vi "Random Graph Generator.vi"() -> ()   [LabVIEW 2021]
panel:
  in  "Array":T1(array[cluster])
  in  "Show Graph?":bool
  in  "Graph Type":enum16{"Velocity", "Position"}(ring)=enum."Position"
  out "Waveform Graph":dbl[][](graph)
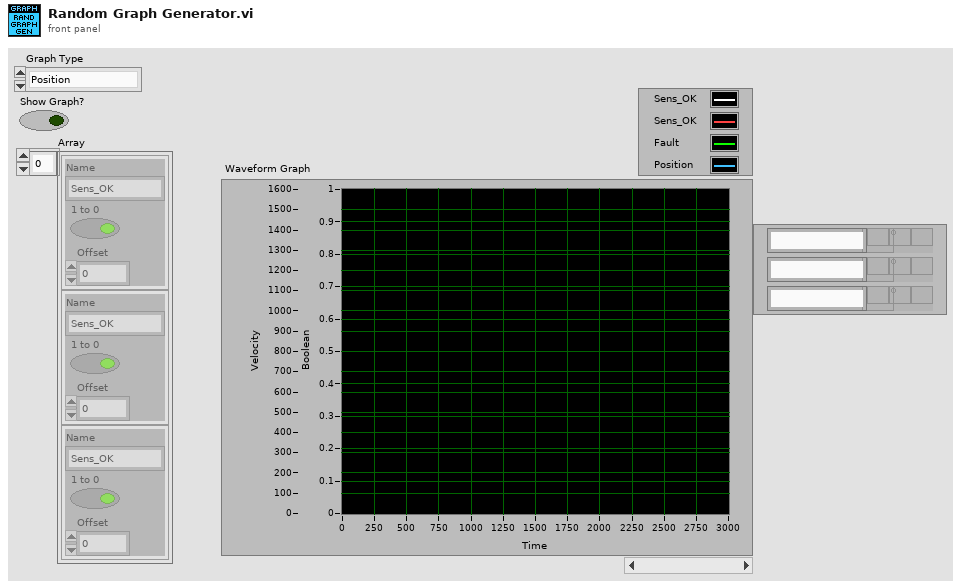
[diagram p1: front panel]
types:
  T1 = cluster{"Name":string, "1 to 0":bool, "Offset":dbl}[]
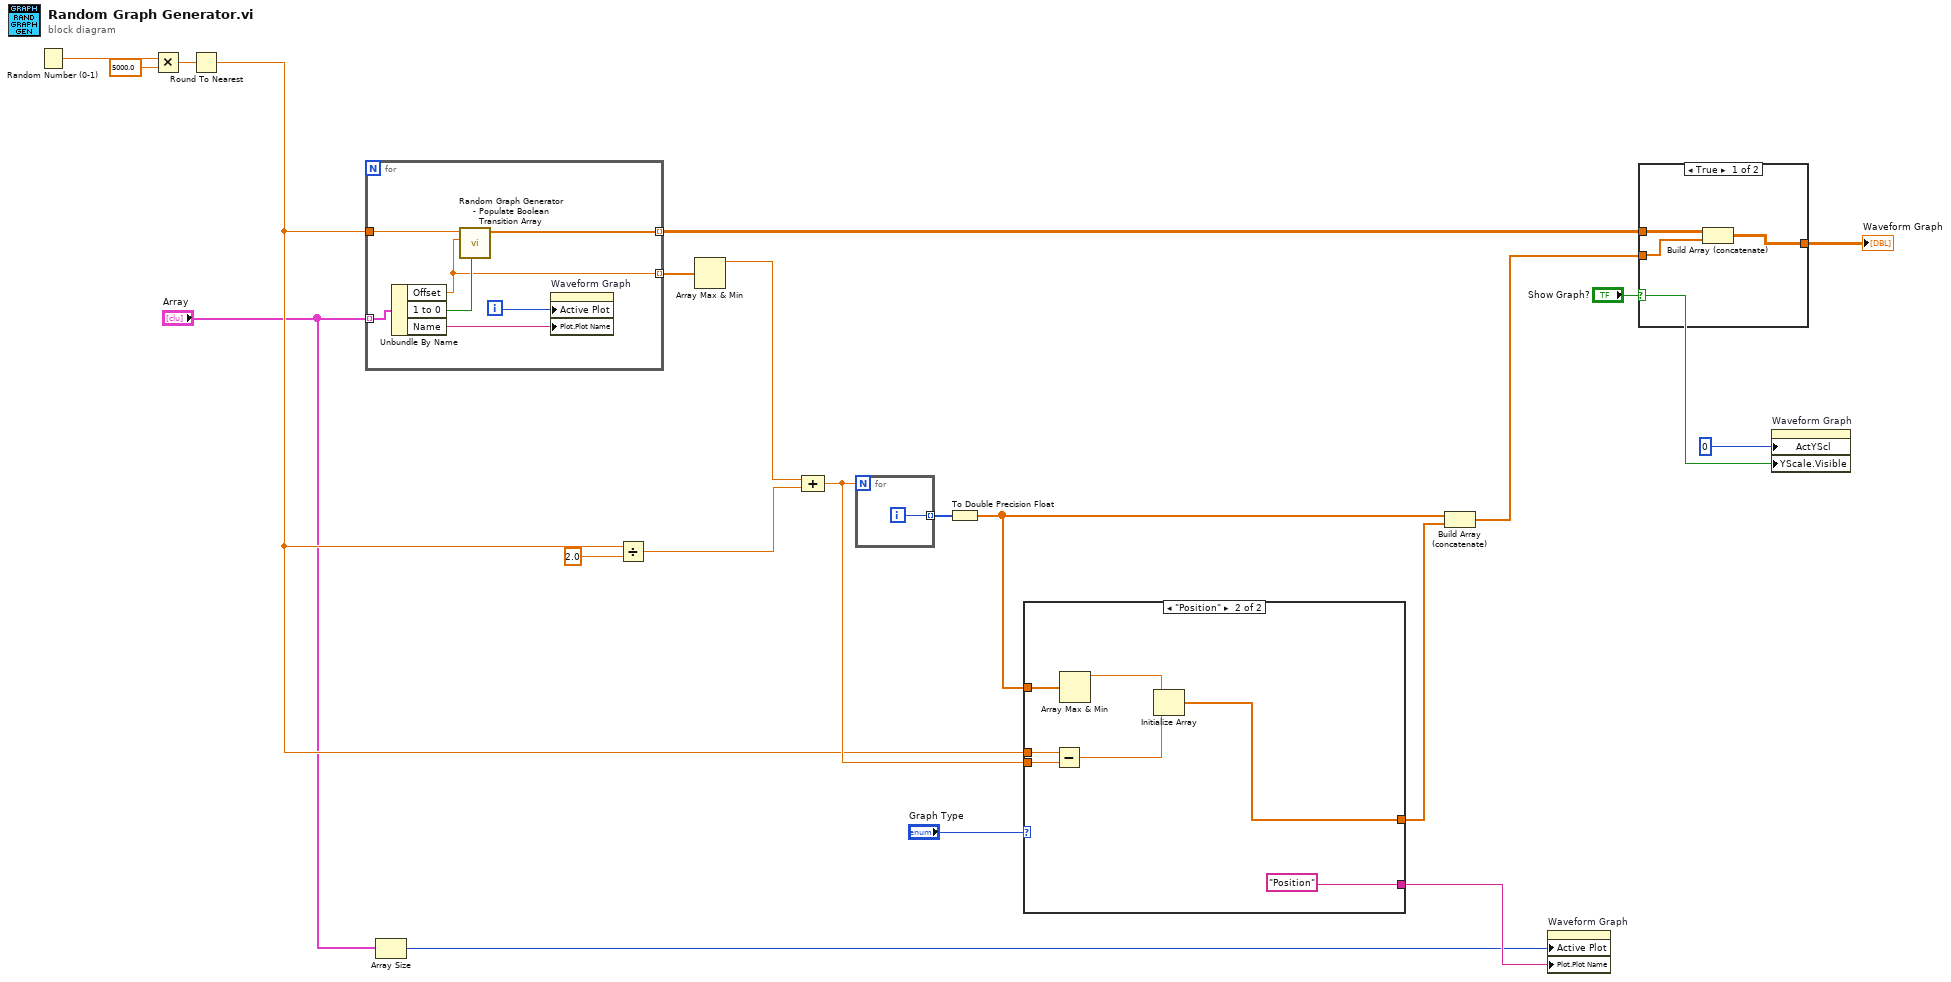
[diagram p0: block diagram]
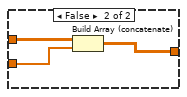
[diagram p2: hidden frame]
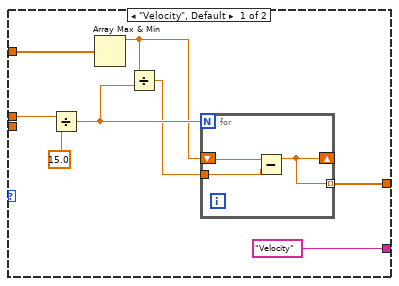
[diagram p3: hidden frame]
diagram:
  n1 = Random Number (0-1)() -> (number: 0 to 1=w21:dbl)
  n2 = Multiply(x=w21, y=5000.0) -> (x*y=w19:dbl)
  n3 = Round To Nearest(number=w19) -> (nearest integer value=w6:dbl)
  n4 = for {
    tunnel: [w28] -> w7 mode=indexing
    tunnel: "Array" -> [w26] mode=indexing
    tunnel: w6 -> [w27]
    tunnel: [w22] -> w5 mode=indexing
    i -> [w24]
    n5 = Unbundle By Name(w26) -> ("Offset"=w22:dbl, "1 to 0"=w25:bool, "Name"=w23:string)
    n6 = call "Random Graph Generator - Populate Boolean Transition Array.vi"("1 to 0"=w25, "Offset"=w22, "Array Size"=w27) -> ("Array"=w28:dbl[])  [unwired: 8 in]
    n7 = property on="Waveform Graph" class="WFGraph (strict)"("Active Plot"=w24, "Plot.Plot Name"=w23) -> ()  [unwired: 2 in, 2 out]
  }
  n8 = Array Size(array="Array") -> (size(s)=w1:i32)
  n9 = Divide(x=w6, y=2.0) -> (x/y=w16:dbl)
  n10 = Array Max & Min(array=w5) -> (max value=w4:dbl)  [unwired: 3 out]
  n11 = Compound Arithmetic op=ADD(w4, w16) -> (w11:dbl)
  n12 = for {
    N: w11 -> [_]
    tunnel: [w29] -> w15 mode=indexing
    i -> [w29]
  }
  n13 = To Double Precision Float(number=w15) -> (double precision float=w8:dbl[])
  n14 = case shown="\"Position\"" "Graph Type" {
    tunnel: w6 -> [w37 w47]
    tunnel: w8 -> [w32 w45]
    tunnel: [w31 w42] -> w13
    tunnel: w11 -> [_ w46]
    tunnel: ["Velocity" ("Plot.Plot Name") "Position" ("Plot.Plot Name")] -> w2
    frame "Velocity", Default {
      n15 = Divide(x=w37, y=15.0) -> (x/y=w35:dbl)
      n16 = Array Max & Min(array=w32) -> (max value=w34:dbl)  [unwired: 3 out]
      n17 = Divide(x=w34, y=w35) -> (x/y=w33:dbl)
      n18 = for {
        N: w35 -> [_]
        shift-right: [w38] -> _
        shift-left: w34 -> [w40]
        tunnel: w33 -> [w39]
        tunnel: [w38] -> w31 mode=indexing
        n19 = Subtract(x=w40, y=w39) -> (x-y=w38:dbl)
      }
    }
    frame "Position" {
      n20 = Subtract(x=w47, y=w46) -> (x-y=w43:dbl)
      n21 = Array Max & Min(array=w45) -> (max value=w44:dbl)  [unwired: 3 out]
      n22 = Initialize Array(w44, w43) -> (w42:dbl[])
    }
  }
  n23 = Build Array (concatenate)(w8, w13) -> (w14:dbl[])
  n24 = property on="Waveform Graph" class="WFGraph (strict)"("Active Plot"=w1, "Plot.Plot Name"=w2) -> ()  [unwired: 2 in, 2 out]
  n25 = case shown="True" "Show Graph?" {
    tunnel: w7 -> [w50 w53]
    tunnel: [w49 w52] -> w18
    tunnel: w14 -> [w48 w51]
    frame True {
      n26 = Build Array (concatenate)(w50, w48) -> (w49:dbl[][])
    }
    frame False {
      n27 = Build Array (concatenate)(w53, w51) -> (w52:dbl[][])
    }
  }
  "Waveform Graph" <- w18
  n28 = property on="Waveform Graph" class="WFGraph (strict)"("ActYScl"=0 ("Active Y Scale"), "YScale.Visible"="Show Graph?") -> ()  [unwired: 2 in, 2 out]
